vi "system calibration.vi"(0 "temperature from calibrator":dbl=555.0 format="%.2f", 2 "Calibrator and LV acquired data":dbl[][](array[numeric])=[[0.0, 0.11999999731779099], [5.0, 5.039999961853027], [10.0, 10.069999694824219], [15.0, 15.100000381469727], [20.0, 20.09000015258789], [25.0, 25.1200008392334], [30.0, 30.1200008392334], [40.0, 40.16999816894531], [60.0, 60.16999816894531], [80.0, 80.12000274658203], [100.0, 100.12999725341797], [150.0, 150.2100067138672], [200.0, 200.16000366210938], [250.0, 250.22999572753906], [300.0, 300.239990234375], [350.0, 350.1700134277344], [400.0, 400.20001220703125], [450.0, 450.17999267578125], [500.0, 500.1400146484375], [550.0, 550.22998046875], [600.0, 600.1900024414062], [650.0, 650.2000122070312], [700.0, 700.219970703125], [750.0, 750.219970703125], [800.0, 800.25], [850.0, 850.280029296875], [900.0, 900.3300170898438], [950.0, 950.280029296875], [1000.0, 1000.3099975585938], [1050.0, 1050.2900390625], [1100.0, 1100.3299560546875], [1112.0, 1112.3900146484375], [1120.0, 1120.4100341796875], [1125.0, 1125.4100341796875]] format="%.3f", 4 "algorithm":T1(ring)=enum."Givens", 5 "polynomial order":i32=3) -> (6 "LabVIEW calculated value using poly fit":dbl=777.0803608582349 format="%.2f")   [LabVIEW 2010]
doc: "Interpolates the function f at x, given a set of n points {x(i),y(i)} where f(x(i))=y(i), f is any function and x is in the range of x(i).\nThe VI caculates output interpolation value Pn-1(x), where Pn-1 is the unique polynomial of degree n-1 that passes through the n points{x(i),y(i)}."
uses:
  <vilib>/Analysis/NI_AALPro.lvlib
panel:
  # "This VI takes a 2d array where first column is the Fluke cal data, the second acquired data measure by LabVIEW.\nTemperature from calibrator is the value you input from your calibrated source.\nLabVIEW calculated calue using poly fit is the value LV measures."
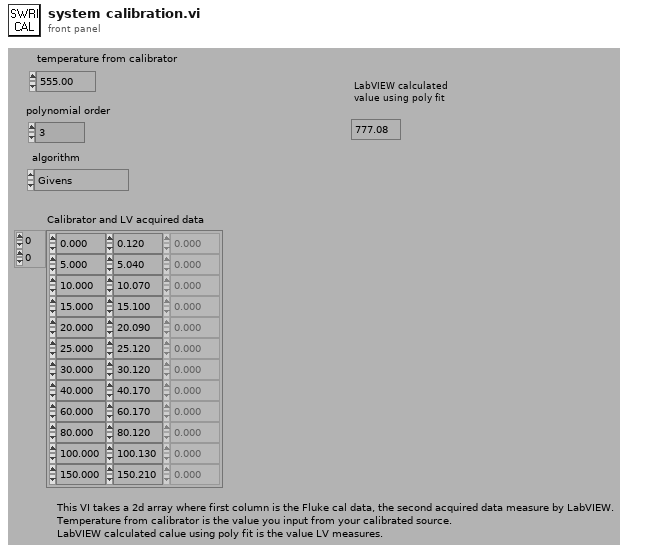
[diagram p1: front panel]
types:
  T1 = enum32{"SVD", "Givens", "Givens2", "Householder", "LU Decomposition", "Cholesky"}
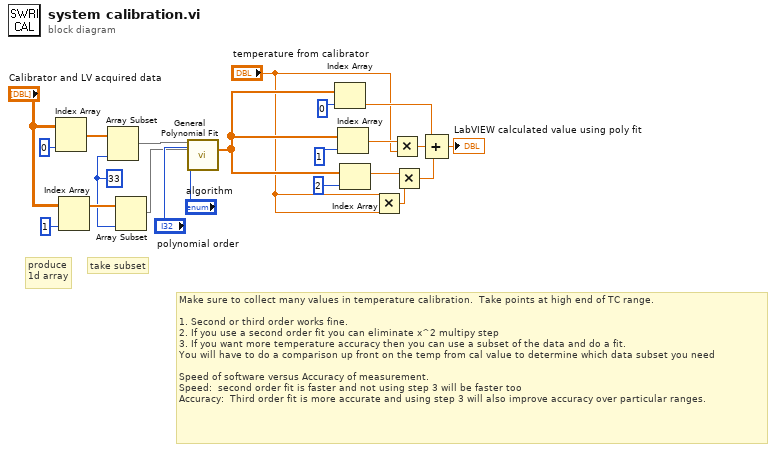
[diagram p0: block diagram]
diagram:
  w4 = 33 ("Array Length")
  # "Make sure to collect many values in temperature calibration.  Take points at high end of TC range.\n\n1. Second or third order works fine.\n2. If you use a second order fit you can eliminate x^2 multipy step\n3. If you want more temperature accuracy then you can use a subset of the data and do a fit.  \nYou will have to do a comparison up front on the temp from cal value to determine which data subset you need\n\nSpeed of software versus Accuracy of measurement.\nSpeed:  second order fit is faster and not using step 3 will be faster too\nAccuracy:  Third order fit is more accurate and using step 3 will also improve accuracy over particular ranges."
  # "take subset"
  # "produce\n1d array"
  n1 = Index Array(array="Calibrator and LV acquired data", index (col)=0 ("Index")) -> (element=w6:dbl[])  [unwired: 1 in]
  n2 = Index Array(array="Calibrator and LV acquired data", index (col)=1 ("Index")) -> (element=w5:dbl[])  [unwired: 1 in]
  n3 = Array Subset(array=w6, length=w4) -> (w1:dbl[])  [unwired: 1 in]
  n4 = Array Subset(array=w5, length=w4) -> (w10:dbl[])  [unwired: 1 in]
  n5 = call <vilib>:"General Polynomial Fit.vi"("Y"=w1, "polynomial order"="polynomial order", "X"=w10, "algorithm"="algorithm") -> ("Polynomial Coefficients"=w3:dbl[])  [unwired: 8 in, 3 out]
  n6 = Index Array(array=w3, index=0 ("Disabled Index")) -> (element=w16:dbl)
  n7 = Index Array(array=w3, index=1 ("Disabled Index")) -> (element=w17:dbl)
  n8 = Index Array(array=w3, index=2 ("Disabled Index")) -> (element=w13:dbl)
  n9 = Multiply(x="temperature from calibrator", y="temperature from calibrator") -> (x*y=w12:dbl)
  n10 = Multiply(x=w17, y="temperature from calibrator") -> (x*y=w15:dbl)
  n11 = Multiply(x=w13, y=w12) -> (x*y=w14:dbl)
  n12 = Compound Arithmetic op=ADD(w16, w15, w14) -> (→"LabVIEW calculated value using poly fit":dbl)
